vi "Current Tool.vi"(7 "Get/Set":enum16{"Get", "Set"}(ring), 8 "error in (no error)":errorcluster, 9 "Tool in":string, 11 "FlexWorktable in":refnum<class "FlexWorktable.lvclass">) -> (0 "error out":errorcluster, 1 "Tool out":string, 3 "FlexWorktable out":refnum<class "FlexWorktable.lvclass">, 5 "Rack Position":i32)   [LabVIEW 2017, in "FlexWorktable.lvclass"]
uses:
  FlexWorktable.lvclass
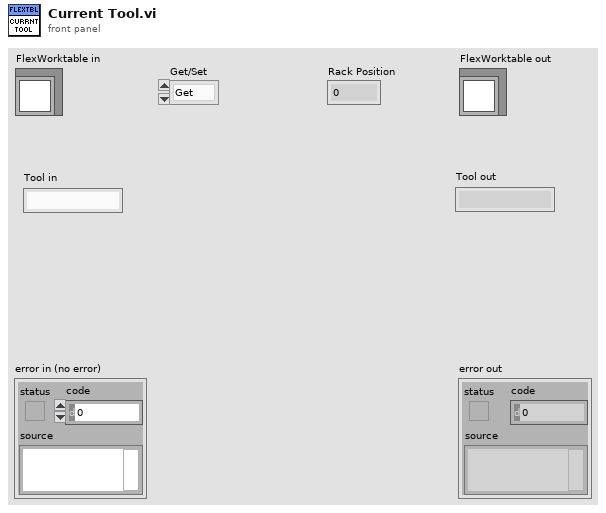
[diagram p1: front panel]
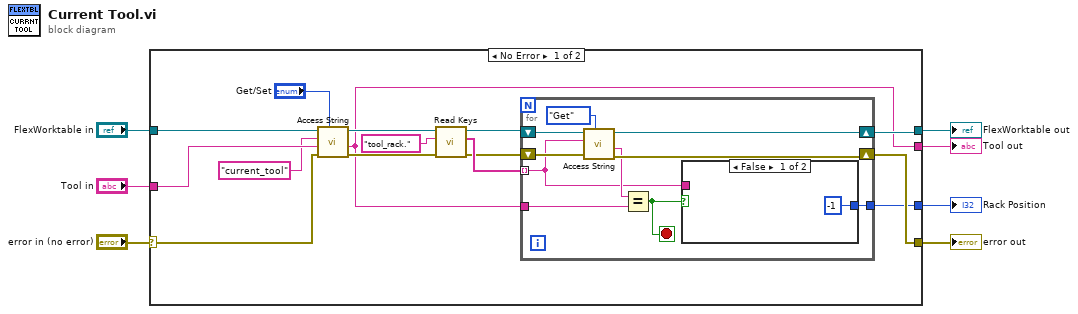
[diagram p0: block diagram]
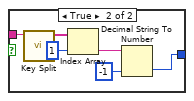
[diagram p2: hidden frame]
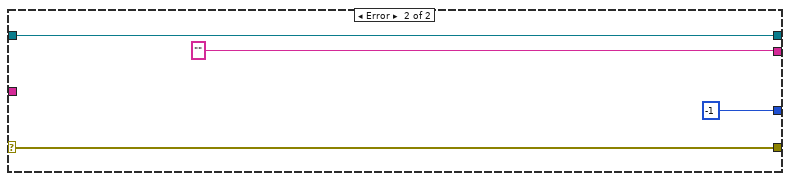
[diagram p3: hidden frame]
diagram:
  n1 = case shown="No Error" "error in (no error)" {
    selector: "error in (no error)" -> [w20 w43]
    tunnel: [w9 w43] -> w6
    tunnel: [w11 w42] -> w4
    tunnel: "FlexWorktable in" -> [w21 w42]
    tunnel: "Tool in" -> [w22 _]
    tunnel: [w10 "" ("Value out")] -> w2
    tunnel: [w8 -1] -> w1
    frame No Error {
      n2 = call-dynamic "Access String.vi"("Get/Set"="Get/Set", "error in (no error)"=w20, "Value in"=w22, "Key"="current_tool", "FlexWorktable in"=w21) -> ("error out"=w15:errorcluster, "Value out"=w10:string, "FlexWorktable out"=w17:refnum<class "FlexWorktable.lvclass">)  [unwired: 4 in]
      n3 = call-dynamic "Read Keys.vi"("error in (no error)"=w15, "Selector"="tool_rack.", "FlexWorktable in"=w17) -> ("error out"=w12:errorcluster, "Keys"=w13:string[], "FlexWorktable out"=w14:refnum<class "FlexWorktable.lvclass">)  [unwired: 6 in]
      n4 = for {
        tunnel: w13 -> [w25] mode=indexing
        shift-right: [w31] -> w11
        shift-left: w14 -> [w32]
        shift-right: [w28] -> w9
        shift-left: w12 -> [w29]
        tunnel: w10 -> [w26]
        tunnel: [w24] -> w8
        stop <- w23 stop-if-true
        n5 = call-dynamic "Access String.vi"("Get/Set"=enum16{"Get", "Set"}."Get", "error in (no error)"=w29, "Key"=w25, "FlexWorktable in"=w32) -> ("error out"=w28:errorcluster, "Value out"=w27:string, "FlexWorktable out"=w31:refnum<class "FlexWorktable.lvclass">)  [unwired: 5 in]
        n6 = Equal?(x=w27, y=w26) -> (x = y?=w23:bool)
        n7 = case shown="False" w23 {
          tunnel: w25 -> [_ w39]
          tunnel: [-1 w35] -> w24
          frame False {
          }
          frame True {
            n8 = call "Key Split.vi"("Key"=w39) -> ("Key Elements"=w38:string[])  [unwired: 10 in]
            n9 = Index Array(array=w38, index=1) -> (element=w36:string)
            n10 = Decimal String To Number(string=w36, default (0L)=-1 ("default (0 I32)")) -> (number=w35:i32)  [unwired: 1 in, 1 out]
          }
        }
      }
    }
    frame Error {
    }
  }
  "error out" <- w6
  "FlexWorktable out" <- w4
  "Tool out" <- w2
  "Rack Position" <- w1
